vi "Generic command handler.vi"(8 "error in (no error)":errorcluster, 10 "Message in":refnum<class "GenericMessage.lvclass">, 11 "RSA in":refnum<class "RSA.lvclass">) -> (0 "error out":errorcluster, 2 "command":string, 3 "RSA out":refnum<class "RSA.lvclass">)   [LabVIEW 2012, in "RSA.lvclass"]
doc: "The generic_command_handler processes the command 'generic'. Commands which are not part of the predefined list of commands fall under the 'generic' command for special activity."
uses:
  RSA.lvclass
  <vilib>/Distrio/Murmex/GenericMessage/GenericMessage.lvclass
  <vilib>/Distrio/Murmex/Murmex/Murmex.lvclass
  RSA.lvclass/RSA.ctl
  <vilib>/Analysis/NI_AALBase.lvlib
panel:
  # "This method is called when the GENERIC\ntrigger is sent. \n\nOverride this method when your component needs to\nrespond to this trigger. \n\nCall parent for proper implementation"
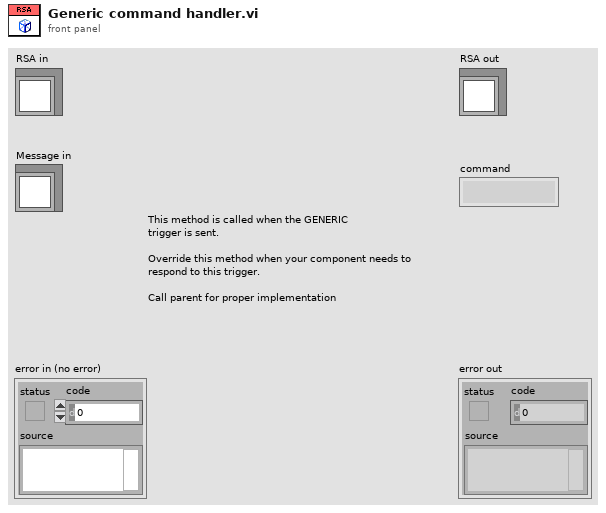
[diagram p1: front panel]
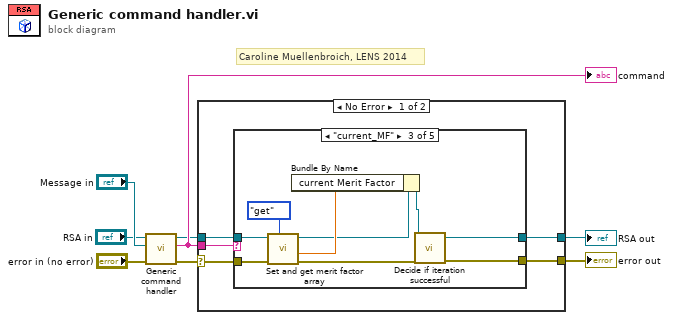
[diagram p0: block diagram]
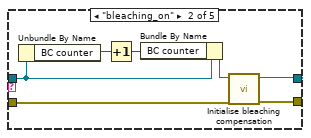
[diagram p3: hidden frame]
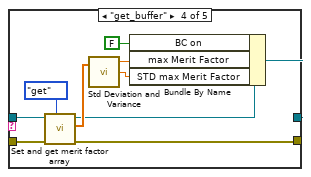
[diagram p4: hidden frame]
diagram:
  # "Caroline Muellenbroich, LENS 2014"
  n1 = call-parent "Generic command handler.vi"("error in (no error)"="error in (no error)", "Message in"="Message in", "Murmex in"="RSA in") -> ("error out"=w5:errorcluster, "value"=w4:string, "Murmex out"=w2:refnum<class "RSA.lvclass">)  [unwired: 6 in]
  "command" <- w4
  n2 = case shown="No Error" w5 {
    selector: w5 -> [w13 w45]
    tunnel: w4 -> [w12 _]
    tunnel: [w11 w45] -> w3
    tunnel: w2 -> [w10 w44]
    tunnel: [w9 w44] -> w1
    frame No Error {
      n3 = case shown="\"current_MF\"" w12 {
        tunnel: w13 -> [w15 w22 w30 w36 w42]
        tunnel: [w15 w21 w25 w34 w42] -> w11
        tunnel: w10 -> [w14 w20 w29 w35 w43]
        tunnel: [w14 w18 w23 w32 w43] -> w9
        frame "False", Default {
        }
        frame "bleaching_on" {
          n4 = Unbundle By Name(w20) -> ("BC counter"=w17:i32)
          n5 = Increment(x=w17) -> (x+1=w16:i32)
          n6 = Bundle By Name(cluster=w20, "BC counter"=w16) -> (w19:refnum<class "RSA.lvclass">)
          n7 = call-dynamic "Initialise bleaching compensation.vi"("error in (no error)"=w22, "RSA in"=w19) -> ("error out"=w21:errorcluster, "RSA out"=w18:refnum<class "RSA.lvclass">)  [unwired: 8 in]
        }
        frame "current_MF" {
          n8 = call "Set and get merit factor array.vi"("action"=enum16{"set", "get", "initialise"}."get", "error in (no error)"=w30, "RSA in"=w29) -> ("error out"=w26:errorcluster, "current merit factor"=w28:dbl, "RSA out"=w27:refnum<class "RSA.lvclass">)  [unwired: 5 in, 1 out]
          n9 = Bundle By Name(cluster=w27, "current Merit Factor"=w28) -> (w24:refnum<class "RSA.lvclass">)
          n10 = call-dynamic "Decide if iteration successful.vi"("error in (no error)"=w26, "RSA in"=w24) -> ("error out"=w25:errorcluster, "RSA out"=w23:refnum<class "RSA.lvclass">)  [unwired: 8 in]
        }
        frame "get_buffer" {
          n11 = call "Set and get merit factor array.vi"("action"=enum16{"set", "get", "initialise"}."get", "error in (no error)"=w36, "RSA in"=w35) -> ("error out"=w34:errorcluster, "merit factor array"=w40:dbl[], "RSA out"=w33:refnum<class "RSA.lvclass">)  [unwired: 5 in, 1 out]
          n12 = call <vilib>:"Std Deviation and Variance.vi"("X"=w40) -> ("mean"=w37:dbl, "standard deviation"=w38:dbl)  [unwired: 1 in, 1 out]
          n13 = Bundle By Name(cluster=w33, "BC on"=FALSE ("Run time cluster.BC on"), "max Merit Factor"=w37, "STD max Merit Factor"=w38) -> (w32:refnum<class "RSA.lvclass">)
        }
        frame "dummy" {
        }
      }
    }
    frame Error {
    }
  }
  "error out" <- w3
  "RSA out" <- w1
